vi "Collect Scaffold Refs.vi"(11 "Class Item":refnum<vi>) -> (3 "Scaffold Project Refs":T1)   [LabVIEW 2018, in "LVClassByRef.lvlib"]
uses:
  <resource>/Framework/Providers/LVClassByRef/LVClassByRef.lvlib
  <resource>/Framework/Providers/LVClassByRef/Scaffold Project Refs.ctl
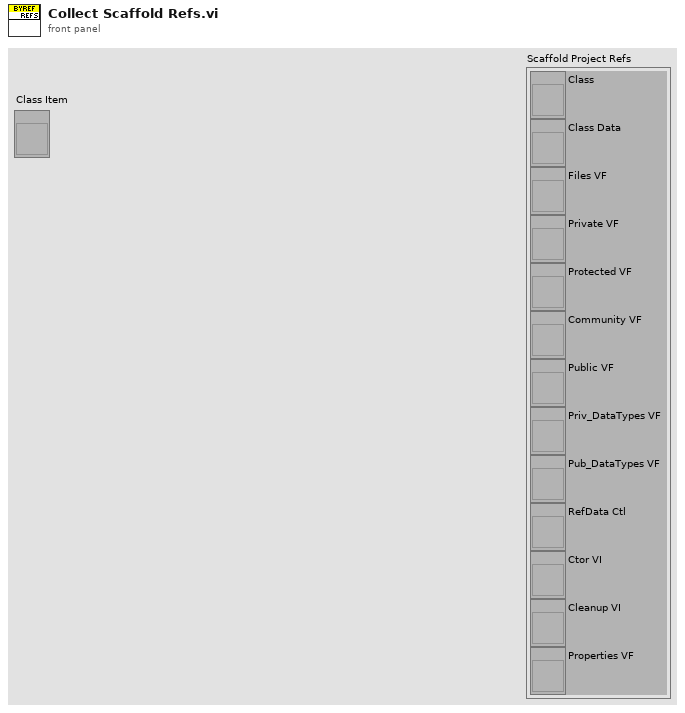
[diagram p1: front panel]
types:
  T1 = typedef "LVClassByRef.lvlib/Scaffold Project Refs.ctl" = cluster{"Class":refnum<vi>, "Class Data":refnum<vi>, "Files VF":refnum<vi>, "Private VF":refnum<vi>, "Protected VF":refnum<vi>, "Community VF":refnum<vi>, "Public VF":refnum<vi>, "Priv_DataTypes VF":refnum<vi>, "Pub_DataTypes VF":refnum<vi>, "RefData Ctl":refnum<vi>, "Ctor VI":refnum<vi>, "Cleanup VI":refnum<vi>, "Properties VF":refnum<vi>}
  T2 = typedef "LVClassByRef.lvlib/Enumerated Item.ctl" = cluster{"Item":refnum<vi>, "Library":refnum<vi>}
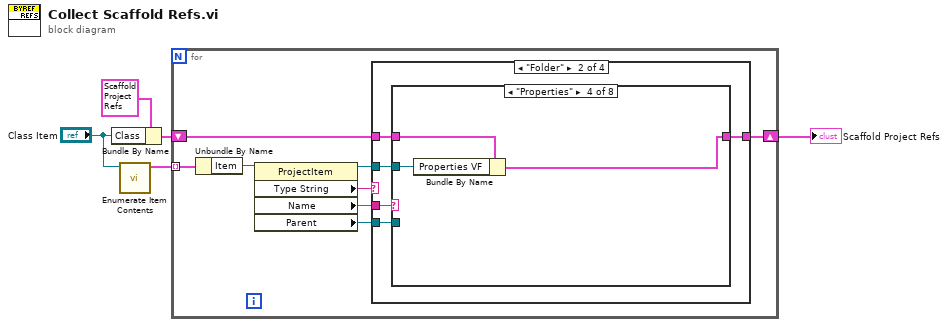
[diagram p0: block diagram]
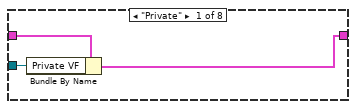
[diagram p3: hidden frame]
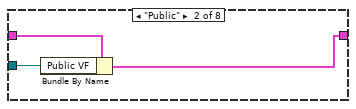
[diagram p4: hidden frame]
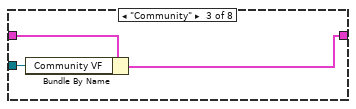
[diagram p5: hidden frame]
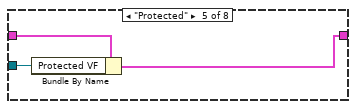
[diagram p6: hidden frame]
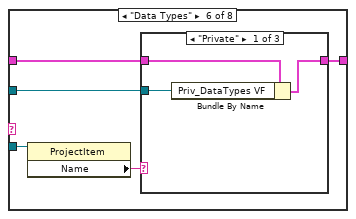
[diagram p7: hidden frame]
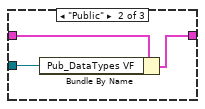
[diagram p8: hidden frame]
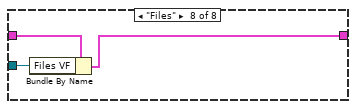
[diagram p11: hidden frame]
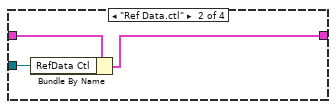
[diagram p13: hidden frame]
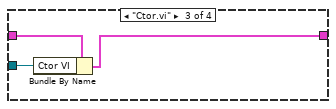
[diagram p14: hidden frame]
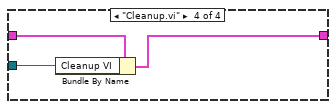
[diagram p15: hidden frame]
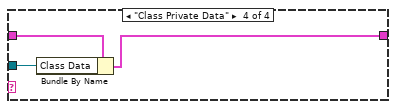
[diagram p16: hidden frame]
diagram:
  n1 = Bundle By Name(cluster=T1 {"Class"=refnum, "Class Data"=refnum, "Files VF"=refnum, "Private VF"=refnum, "Protected VF"=refnum, "Community VF"=refnum, "Public VF"=refnum, "Priv_DataTypes VF"=refnum, "Pub_DataTypes VF"=refnum, "RefData Ctl"=refnum, "Ctor VI"=refnum, "Cleanup VI"=refnum, "Properties VF"=refnum} ("Scaffold Project Refs"), "Class"="Class Item") -> (w4:T1)
  n2 = call <resource>:"Enumerate Item Contents.vi"("ProjectItem Refnum"="Class Item") -> ("Nested Items"=w3:T2[])  [unwired: 10 in]
  n3 = for {
    shift-right: [w9] -> w1
    shift-left: w4 -> [w11]
    tunnel: w3 -> [w7] mode=indexing
    n4 = Unbundle By Name(w7) -> ("Item"=w6:refnum<vi>)
    n5 = property class="ProjectItem"(reference=w6) -> (reference out=w12:refnum<vi>, "Type String"=w13:string, "Name"=w10:string, "Parent"=w8:refnum<vi>)  [unwired: 1 in, 1 out]
    n6 = case shown="\"Folder\"" w13 {
      tunnel: w12 -> [_ w17 w52 w66]
      tunnel: w11 -> [w14 w18 w53 w67]
      tunnel: w10 -> [_ w19 w54 _]
      tunnel: [w14 w16 w51 w65] -> w9
      tunnel: w8 -> [_ w15 _ _]
      frame Default {
      }
      frame "Folder" {
        n7 = case shown="\"Properties\"" w19 {
          tunnel: w18 -> [w22 w25 w28 w31 w34 w38 w47 w50]
          tunnel: w17 -> [w21 w24 w27 w30 w33 w36 _ w49]
          tunnel: [w20 w23 w26 w29 w32 w35 w47 w48] -> w16
          tunnel: w15 -> [_ _ _ _ _ w39 _ _]
          frame "Private" {
            n8 = Bundle By Name(cluster=w22, "Private VF"=w21) -> (w20:T1)
          }
          frame "Public" {
            n9 = Bundle By Name(cluster=w25, "Public VF"=w24) -> (w23:T1)
          }
          frame "Community" {
            n10 = Bundle By Name(cluster=w28, "Community VF"=w27) -> (w26:T1)
          }
          frame "Properties" {
            n11 = Bundle By Name(cluster=w31, "Properties VF"=w30) -> (w29:T1)
          }
          frame "Protected" {
            n12 = Bundle By Name(cluster=w34, "Protected VF"=w33) -> (w32:T1)
          }
          frame "Data Types" {
            n13 = property class="ProjectItem"(reference=w39) -> ("Name"=w37:string)  [unwired: 1 in, 2 out]
            n14 = case shown="\"Private\"" w37 {
              tunnel: w38 -> [w42 w45 w46]
              tunnel: w36 -> [w41 w44 _]
              tunnel: [w40 w43 w46] -> w35
              frame "Private" {
                n15 = Bundle By Name(cluster=w42, "Priv_DataTypes VF"=w41) -> (w40:T1)
              }
              frame "Public" {
                n16 = Bundle By Name(cluster=w45, "Pub_DataTypes VF"=w44) -> (w43:T1)
              }
              frame Default {
              }
            }
          }
          frame Default {
          }
          frame "Files" {
            n17 = Bundle By Name(cluster=w50, "Files VF"=w49) -> (w48:T1)
          }
        }
      }
      frame "VI" {
        n18 = case shown="Default" w54 {
          tunnel: w53 -> [w55 w58 w61 w64]
          tunnel: w52 -> [_ w57 w60 w63]
          tunnel: [w55 w56 w59 w62] -> w51
          frame Default {
          }
          frame "Ref Data.ctl" {
            n19 = Bundle By Name(cluster=w58, "RefData Ctl"=w57) -> (w56:T1)
          }
          frame "Ctor.vi" {
            n20 = Bundle By Name(cluster=w61, "Ctor VI"=w60) -> (w59:T1)
          }
          frame "Cleanup.vi" {
            n21 = Bundle By Name(cluster=w64, "Cleanup VI"=w63) -> (w62:T1)
          }
        }
      }
      frame "Class Private Data" {
        n22 = Bundle By Name(cluster=w67, "Class Data"=w66) -> (w65:T1)
      }
    }
  }
  "Scaffold Project Refs" <- w1
